vi "Parser.vi"() -> ()   [LabVIEW 2014]
panel:
  out "after substring":string
  in  "stop":bool
  out "Match":string
  in  "Input string":string
  in  "Regular expression":string
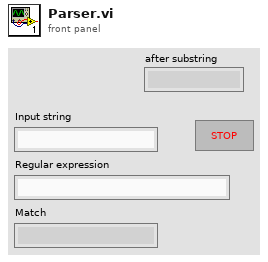
[diagram p1: front panel]
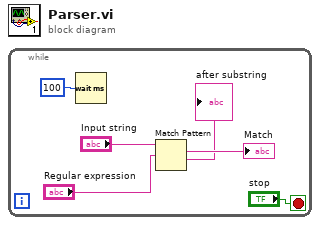
[diagram p0: block diagram]
diagram:
  n1 = while {
    stop <- "stop" stop-if-true
    n2 = Wait (ms)(milliseconds to wait=u32 100) -> ()  [unwired: 1 out]
    n3 = Match Pattern(string="Input string", regular expression="Regular expression") -> (match substring=→"Match":string, after substring=→"after substring":string)  [unwired: 1 in, 2 out]
  }
